vi "WPI_IMU_ADIS16448_SPIDelay.vi"(8 "error in":errorcluster, 10 "Delay (ms)":dbl=100.0 format="%#_13g", 11 "SPIDevRef in":T1) -> (0 "error out":errorcluster, 3 "SPIDevRef out":T1)   [LabVIEW 2015, in "FRC ADI MXP IMU.lvlib"]
uses:
  FRC ADI MXP IMU.lvlib
  <vilib>/Rock Robotics/WPI/SPI/WPI_SPIDevRef.ctl
  <vilib>/Rock Robotics/SystemInterfaces/spilib/spi_bus.ctl
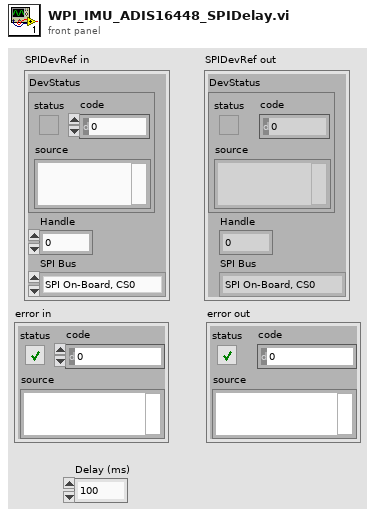
[diagram p1: front panel]
types:
  T1 = typedef "WPI_SPIDevRef.ctl" = cluster{"DevStatus":errorcluster, "Handle":i32, "SPI Bus":T2}
  T2 = typedef "spi_bus.ctl" = enum16{"SPI On-Board, CS0", "SPI On-Board, CS1", "SPI On-Board, CS2", "SPI On-Board, CS3", "SPI MXP", "Invalid"}
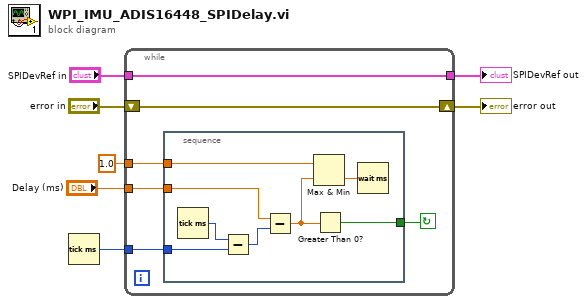
[diagram p0: block diagram]
diagram:
  n1 = Tick Count (ms)() -> (millisecond timer value=w5:u32)
  n2 = while {
    tunnel: "Delay (ms)" -> [w11]
    tunnel: 1.0 -> [w12]
    tunnel: w5 -> [w13]
    tunnel: "SPIDevRef in" -> [w9]
    tunnel: [w9] -> w7
    shift-right: [w8] -> w1
    shift-left: "error in" -> [w8]
    stop <- w10 continue-if-true
    n3 = stacked-sequence {
      tunnel: w13 -> [w21]
      tunnel: w12 -> [w20]
      tunnel: w11 -> [w18]
      tunnel: [w14] -> w10
      frame #0 {
        n4 = Tick Count (ms)() -> (millisecond timer value=w16:u32)
        n5 = Subtract(x=w16, y=w21) -> (x-y=w17:u32)
        n6 = Subtract(x=w18, y=w17) -> (x-y=w15:dbl)
        n7 = Max & Min(x=w20, y=w15) -> (min(x,y)=w19:dbl)  [unwired: 1 out]
        n8 = Greater Than 0?(x=w15) -> (x > 0?=w14:bool)
        n9 = Wait (ms)(milliseconds to wait=w19) -> ()  [unwired: 1 out]
      }
    }
  }
  "SPIDevRef out" <- w7
  "error out" <- w1
